vi "LabVIEW OPC UA Server.vi"() -> ()   [LabVIEW 2020]
uses:
  <vilib>/OPCUA/server/Read Double.vi
  <vilib>/OPCUA/NI OPC UA Server.lvlib
  <vilib>/OPCUA/NI OPC UA Utility.lvlib
panel:
  in  "Settings Button":bool
  out "Running":bool
  in  "Write Button":bool
  out "Items":string[][](table)
  in  "Stop Button":bool
  in  "Start Button":bool
  out "Error out":errorcluster
  in  "Error in":errorcluster
  in  "Exit Button":bool
  out "Server Address":string
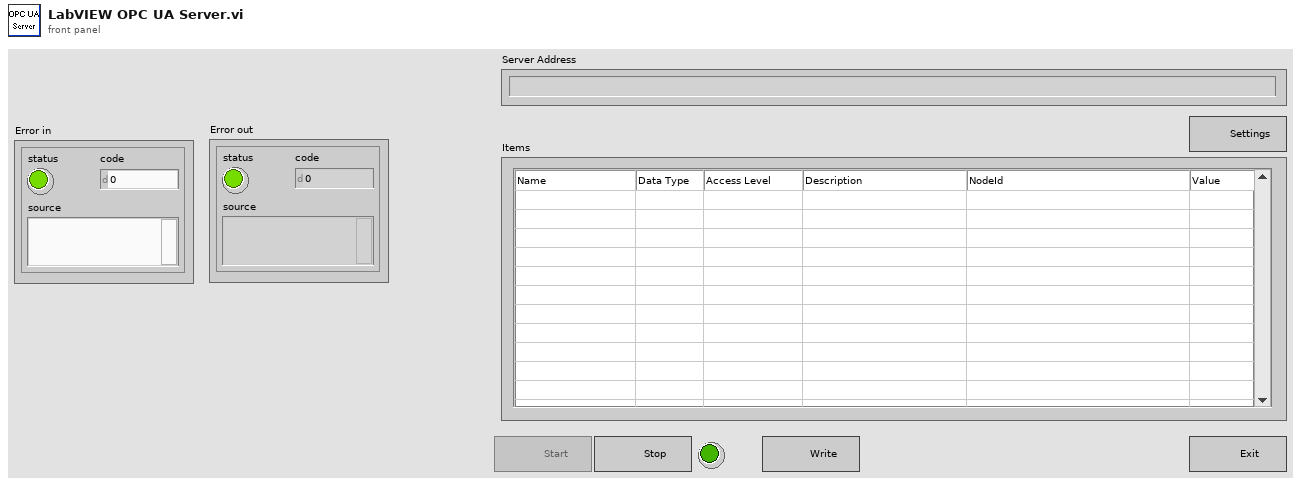
[diagram p1: front panel]
types:
  T1 = enum8{"Enabled", "Disabled", "Disabled and Grayed Out"}
  T2 = typedef "OPC UA Server Refnum.ctl" = refnum<k21>
  T3 = typedef "NodeId.ctl" = string
  T4 = cluster{"Name":string, "Data type":u16, "Access level":u16, "Description":string}[]
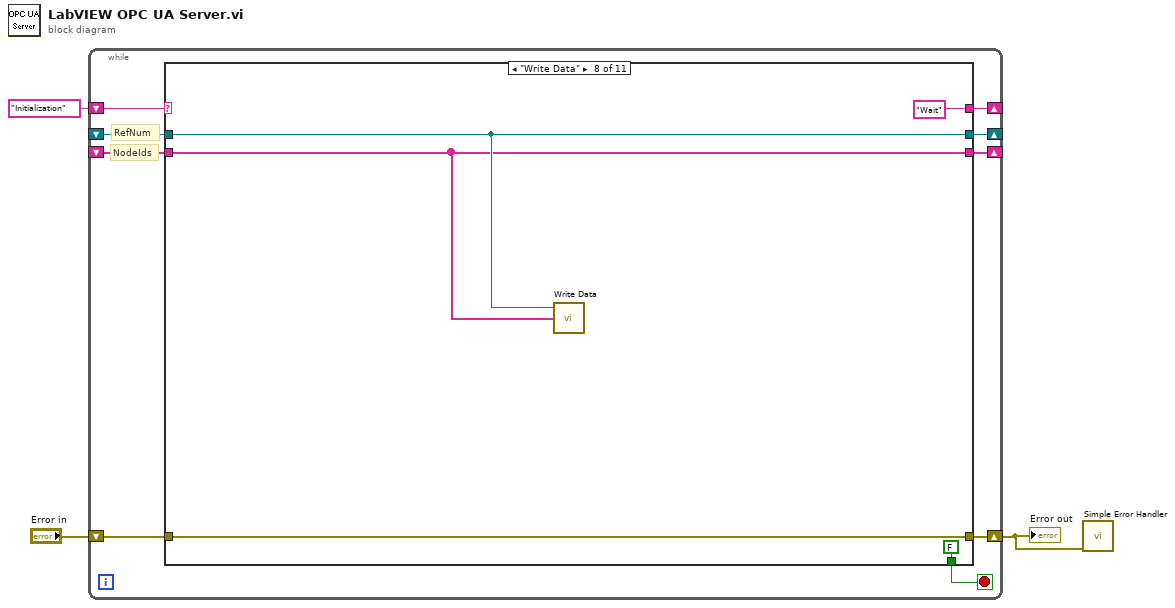
[diagram p0: block diagram]
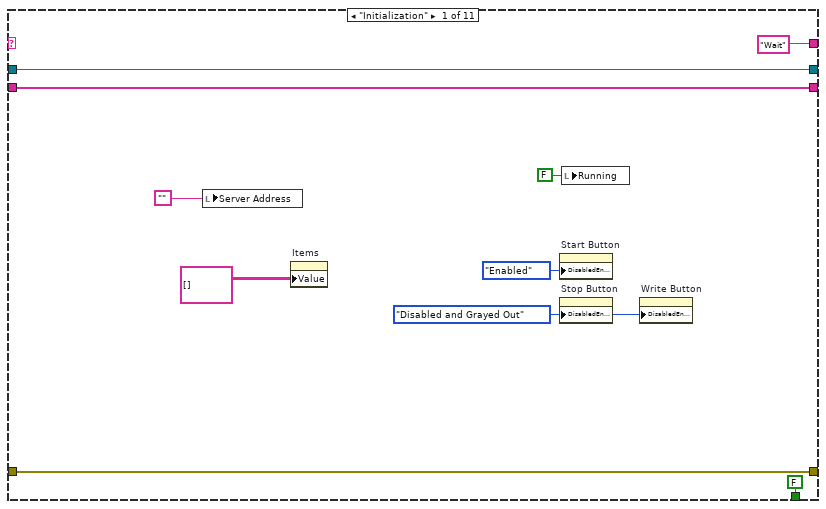
[diagram p2: hidden frame]
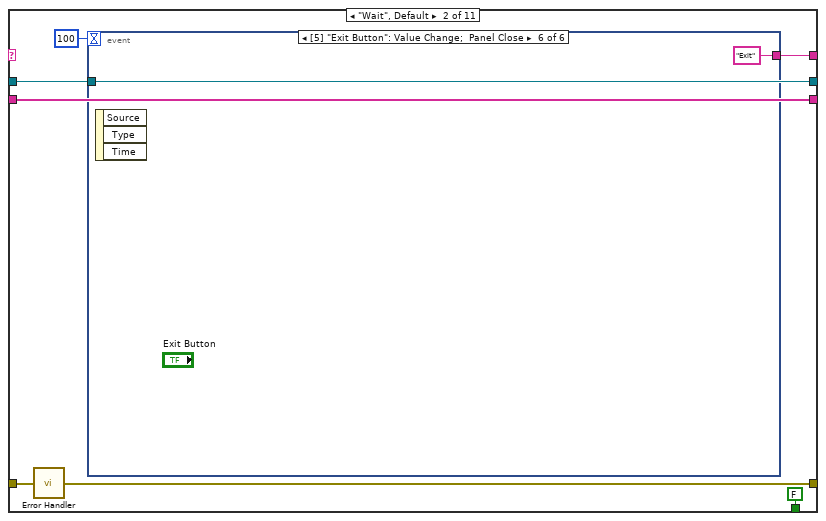
[diagram p3: hidden frame]
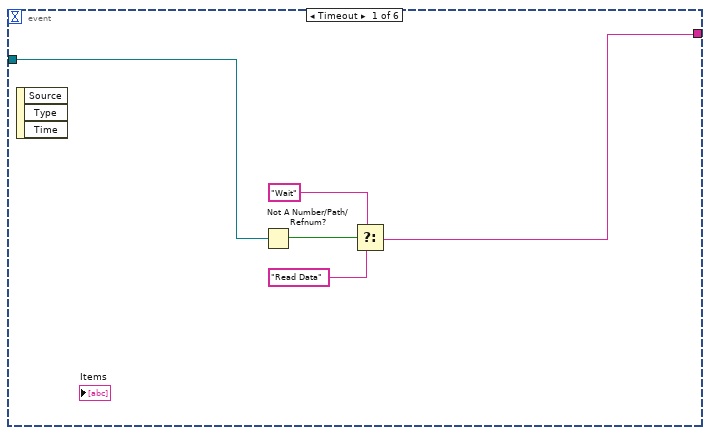
[diagram p4: hidden frame]
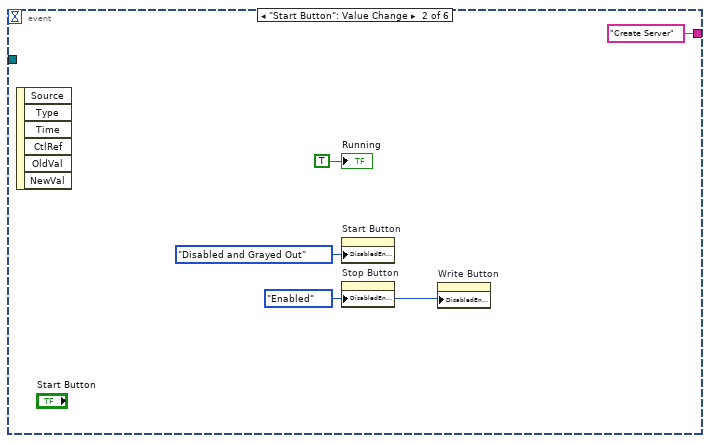
[diagram p5: hidden frame]
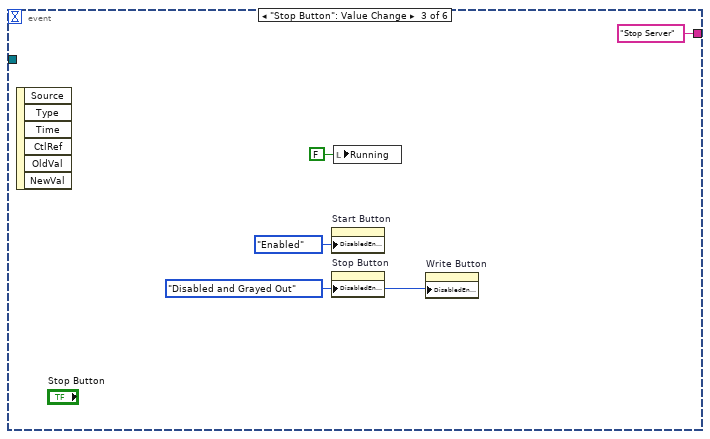
[diagram p6: hidden frame]
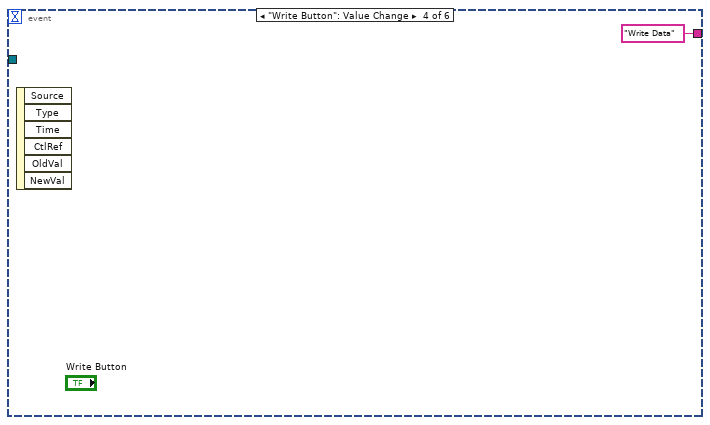
[diagram p7: hidden frame]
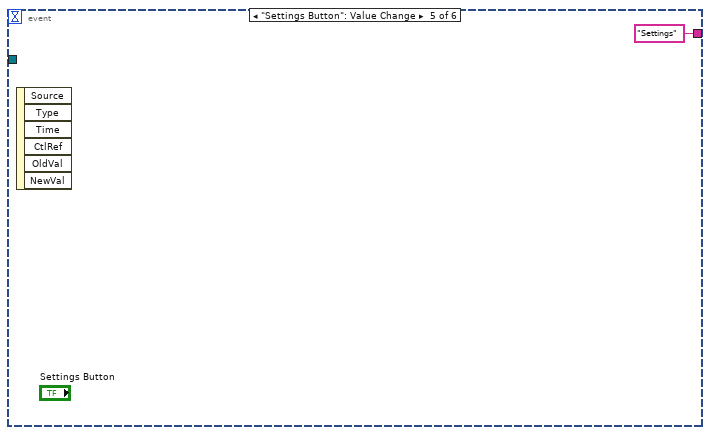
[diagram p8: hidden frame]
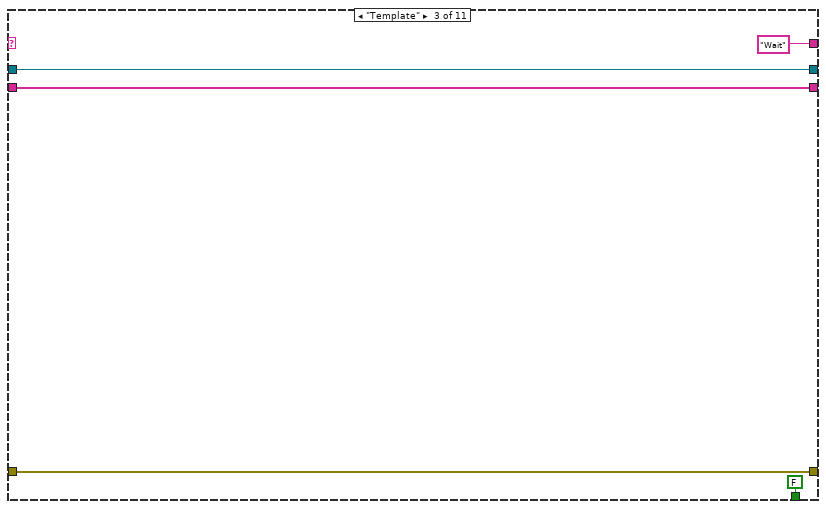
[diagram p9: hidden frame]
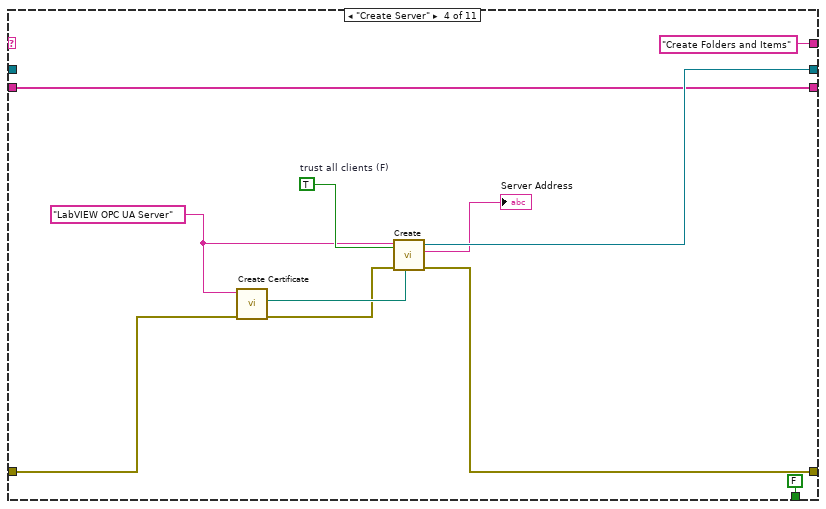
[diagram p10: hidden frame]
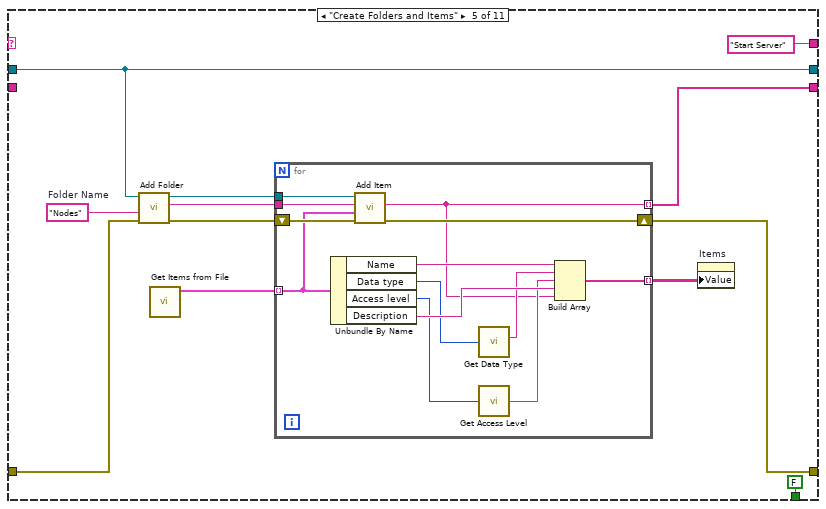
[diagram p11: hidden frame]
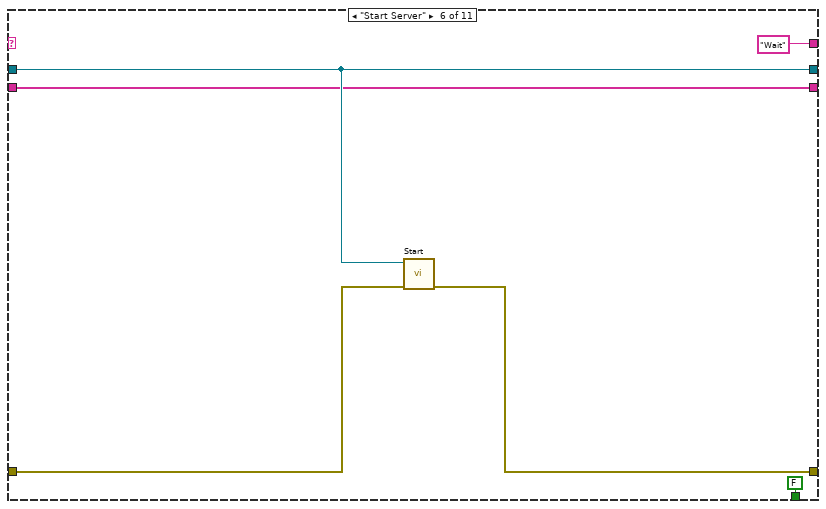
[diagram p12: hidden frame]
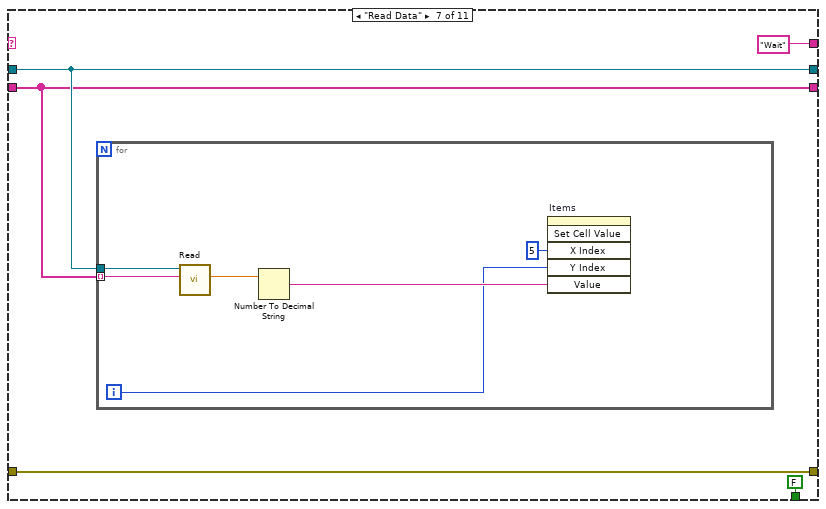
[diagram p13: hidden frame]
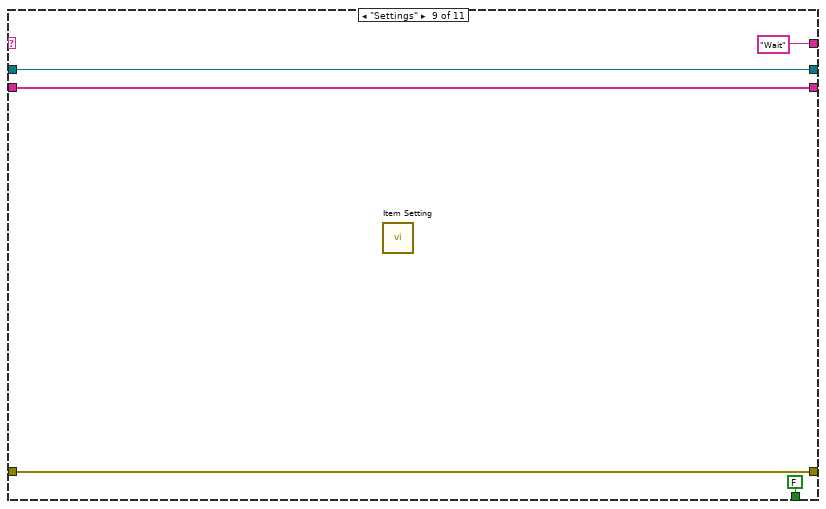
[diagram p14: hidden frame]
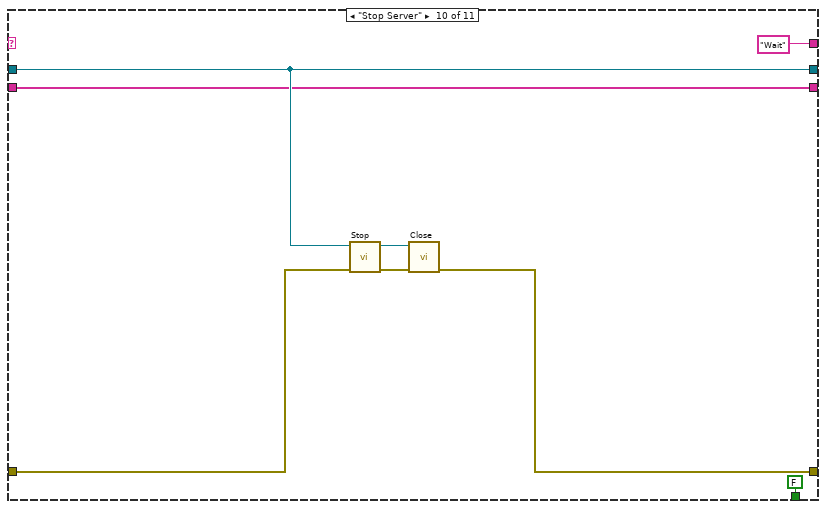
[diagram p15: hidden frame]
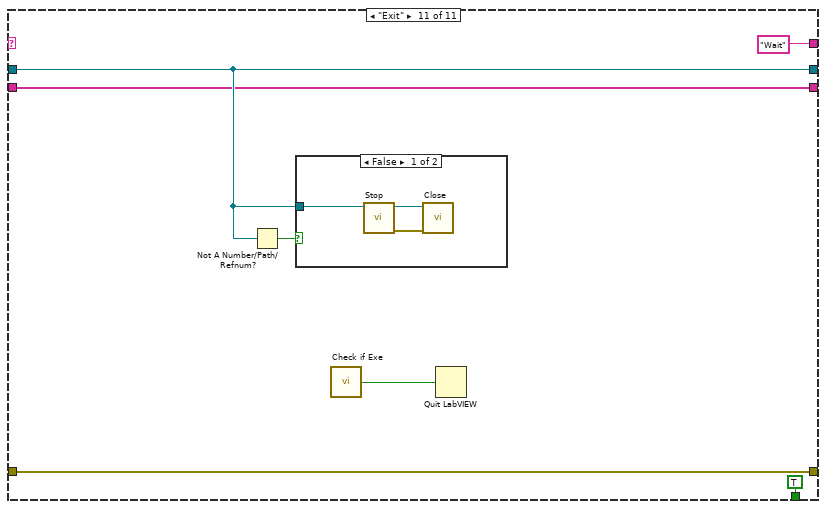
[diagram p16: hidden frame]
diagram:
  n1 = while {
    shift-right: [w11] -> _
    shift-left: "Initialization" -> [w12]
    shift-right: [w9] -> _
    shift-left: _ -> [w8]
    shift-right: [w7] -> w1
    shift-left: "Error in" -> [w6]
    shift-right: [w5] -> _
    shift-left: _ -> [w4]
    stop <- w10 stop-if-true
    # "NodeIds"
    # "RefNum"
    n2 = case shown="\"Write Data\"" w12 {
      tunnel: ["Wait" w29 "Wait" "Create Folders and Items" "Start Server" "Wait" "Wait" "Wait" "Wait" "Wait" "Wait"] -> w11
      tunnel: [FALSE FALSE FALSE FALSE FALSE FALSE FALSE FALSE FALSE FALSE TRUE] -> w10
      tunnel: [w20 w25 w48 w59 w67 w90 w94 w105 w110 w117 w123] -> w9
      tunnel: w8 -> [w20 w25 w48 _ w67 w90 w94 w105 w110 w117 w123]
      tunnel: [w19 w24 w47 w57 w66 w89 w95 w106 w111 w116 w126] -> w7
      tunnel: w6 -> [w19 w23 w47 w53 w65 w88 w95 w106 w111 w115 w126]
      tunnel: [w17 w26 w46 w51 w62 w87 w93 w104 w109 w114 w122] -> w5
      tunnel: w4 -> [w17 w26 w46 w51 _ w87 w93 w104 w109 w114 w122]
      frame "Initialization" {
        w13 = T1."Disabled and Grayed Out" ("Disabled")
        n3 = local write "Server Address"("") -> ()
        n4 = property on="Items" class="Tbl (strict)"("Value"=string[][] [] ("Item Names")) -> ()  [unwired: 2 in, 2 out]
        n5 = property on="Start Button" class="Bool"("DisabledEnum"=T1."Enabled" ("Disabled")) -> ()  [unwired: 2 in, 2 out]
        n6 = property on="Stop Button" class="Bool"("DisabledEnum"=w13) -> ()  [unwired: 2 in, 2 out]
        n7 = local write "Running"(FALSE ("Running")) -> ()
        n8 = property on="Write Button" class="Bool"("DisabledEnum"=w13) -> ()  [unwired: 2 in, 2 out]
      }
      frame "Wait", Default {
        n9 = call "Error Handler.vi"("Error in"=w23) -> ("Error out"=w24:errorcluster)
        n10 = event shown="[5] \"Exit Button\": Value Change;  Panel Close" {
          selector: _ -> [_ _ _ _ _ _]
          dyn-events: _ -> [_ _ _ _ _ _]
          timeout: 100 -> [_ _ _ _ _ _]
          tunnel: [w31 "Create Server" "Stop Server" "Write Data" "Settings" "Exit"] -> w29
          tunnel: w25 -> [w30 _ _ _ _ _]
          event Timeout {
            n11 = event-data() -> ()  [unwired: 1 in, 3 out]
            n12 = Not A Number/Path/Refnum?(number/path/refnum=w30) -> (NaN/Path/Refnum?=w34:bool)
            n13 = Select(t="Wait", s=w34, f="Read Data") -> (s? t:f=w31:string)
          }
          event "Start Button": Value Change {
            w35 = T1."Enabled" ("Disabled")
            n14 = event-data() -> ()  [unwired: 1 in, 6 out]
            n15 = property on="Start Button" class="Bool"("DisabledEnum"=T1."Disabled and Grayed Out" ("Disabled")) -> ()  [unwired: 2 in, 2 out]
            n16 = property on="Stop Button" class="Bool"("DisabledEnum"=w35) -> ()  [unwired: 2 in, 2 out]
            n17 = property on="Write Button" class="Bool"("DisabledEnum"=w35) -> ()  [unwired: 2 in, 2 out]
            "Running" <- TRUE ("Running")
          }
          event "Stop Button": Value Change {
            w39 = T1."Disabled and Grayed Out" ("Disabled")
            n18 = event-data() -> ()  [unwired: 1 in, 6 out]
            n19 = property on="Start Button" class="Bool"("DisabledEnum"=T1."Enabled" ("Disabled")) -> ()  [unwired: 2 in, 2 out]
            n20 = property on="Stop Button" class="Bool"("DisabledEnum"=w39) -> ()  [unwired: 2 in, 2 out]
            n21 = local write "Running"(FALSE ("Running")) -> ()
            n22 = property on="Write Button" class="Bool"("DisabledEnum"=w39) -> ()  [unwired: 2 in, 2 out]
          }
          event "Write Button": Value Change {
            n23 = event-data() -> ()  [unwired: 1 in, 6 out]
          }
          event "Settings Button": Value Change {
            n24 = event-data() -> ()  [unwired: 1 in, 6 out]
          }
          event "Exit Button": Value Change; Panel Close {
            n25 = event-data() -> ()  [unwired: 1 in, 3 out]
          }
        }
      }
      frame "Template" {
      }
      frame "Create Server" {
        w52 = "LabVIEW OPC UA Server" ("certificate name in")
        w56 = TRUE  # trust all clients (F)
        n26 = call <vilib>:"Create Certificate.vi"("error in (no error)"=w53, "certificate name in"=w52) -> ("error out"=w54:errorcluster, "certificate path"=w55:path)  [unwired: 6 in, 2 out]
        n27 = call <vilib>:"Create.vi"("server certificate file"=w55, "trust all clients (F)"=w56, "error in (no error)"=w54, "OPC UA server name"=w52) -> ("error out"=w57:errorcluster, "server endpoint URL"=→"Server Address":string, "OPC UA server refnum out"=w59:T2)  [unwired: 5 in]
      }
      frame "Create Folders and Items" {
        w68 = "Nodes"  # Folder Name
        n28 = call <vilib>:"Add Folder.vi"("error in (no error)"=w65, "folder name"=w68, "OPC UA server refnum in"=w67) -> ("error out"=w69:errorcluster, "folder node ID"=w71:T3, "OPC UA server refnum out"=w70:T2)  [unwired: 5 in]
        n29 = call "Get Items from File.vi"() -> ("Items"=w64:T4)  [unwired: 10 in, 1 out]
        n30 = for {
          tunnel: w71 -> [w86]
          tunnel: w70 -> [w85]
          shift-right: [w83] -> w66
          shift-left: w69 -> [w84]
          tunnel: w64 -> [w82] mode=indexing
          tunnel: [w75] -> w63 mode=indexing
          tunnel: [w74] -> w62 mode=indexing
          n31 = Unbundle By Name(w82) -> ("Name"=w81:string, "Data type"=w79:u16, "Access level"=w77:u16, "Description"=w80:string)
          n32 = call <vilib>:"Add Item.vi"("error in (no error)"=w84, "item"=w82, "parent folder node ID"=w86, "OPC UA server refnum in"=w85) -> ("error out"=w83:errorcluster, "item node ID"=w74:T3)  [unwired: 3 in, 2 out]
          n33 = call "Get Data Type.vi"("Data Type Index"=w79) -> ("Data Type Name"=w78:string)
          n34 = call "Get Access Level.vi"("Access Level Index"=w77) -> ("Access Level Name"=w76:string)
          n35 = Build Array "Build Array"(w81, w78, w76, w80, w74) -> (w75:T3[])
        }
        n36 = property on="Items" class="Tbl (strict)"("Value"=w63) -> ()  [unwired: 2 in, 2 out]
      }
      frame "Start Server" {
        n37 = call <vilib>:"Start.vi"("error in (no error)"=w88, "OPC UA server refnum in"=w90) -> ("error out"=w89:errorcluster)  [unwired: 7 in, 2 out]
      }
      frame "Read Data" {
        n38 = for {
          tunnel: w94 -> [w103]
          tunnel: w93 -> [w102] mode=indexing
          i -> [w98]
          n39 = call-poly <vilib>:"Read.vi"("node ID"=w102, "OPC UA server refnum in"=w103) -> ("value"=w101:dbl)  [unwired: 5 in, 4 out]
          n40 = Number To Decimal String(number=w101) -> (decimal integer string=w100:string)  [unwired: 1 in]
          n41 = invoke on="Items" class="Tbl (strict)" method="Set Cell Value"("X Index"=5, "Y Index"=w98, "Value"=w100) -> ()  [unwired: 3 in, 6 out]
        }
      }
      frame "Write Data" {
        n42 = call "Write Data.vi"("NodeIds"=w104, "OPC UA server refnum"=w105) -> ()  [unwired: 3 in, 1 out]
      }
      frame "Settings" {
        n43 = call "Item Setting.vi"() -> ()  [unwired: 5 in, 1 out]
      }
      frame "Stop Server" {
        n44 = call <vilib>:"Stop.vi"("error in (no error)"=w115, "OPC UA server refnum in"=w117) -> ("error out"=w118:errorcluster, "OPC UA server refnum out"=w119:T2)  [unwired: 8 in]
        n45 = call <vilib>:"Close.vi"("error in (no error)"=w118, "OPC UA server refnum in"=w119) -> ("error out"=w116:errorcluster)  [unwired: 9 in]
      }
      frame "Exit" {
        n46 = Not A Number/Path/Refnum?(number/path/refnum=w123) -> (NaN/Path/Refnum?=w124:bool)
        n47 = case shown="False" w124 {
          tunnel: w123 -> [w129 _]
          frame False {
            n48 = call <vilib>:"Stop.vi"("OPC UA server refnum in"=w129) -> ("error out"=w131:errorcluster, "OPC UA server refnum out"=w130:T2)  [unwired: 9 in]
            n49 = call <vilib>:"Close.vi"("error in (no error)"=w131, "OPC UA server refnum in"=w130) -> ()  [unwired: 9 in, 1 out]
          }
          frame True {
          }
        }
        n50 = call "Check if Exe.vi"() -> ("Executable Application?"=w125:bool)  [unwired: 1 in]
        n51 = Quit LabVIEW(quit? (T)=w125) -> ()
      }
    }
  }
  "Error out" <- w1
  n52 = call <vilib>:"Simple Error Handler.vi"("error in (no error)"=w1) -> ()  [unwired: 4 in, 5 out]
